vi "Interpolate N Between Two Colors.vi"(0 "Starting Color Value":T1, 2 "# Elements":i32=1 min=1, 3 "Ending Color Value":T1) -> (6 "Color Array":T2(array[cluster]))   [LabVIEW 2021, in "Palette.lvlib"]
uses:
  Palette.lvlib
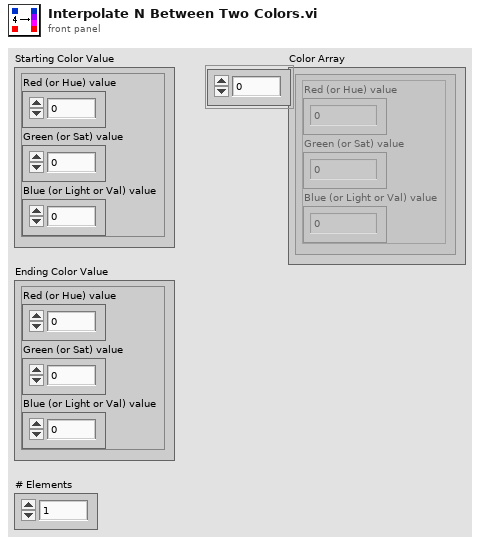
[diagram p1: front panel]
types:
  T1 = cluster{"Red (or Hue) value":u8, "Green (or Sat) value":u8, "Blue (or Light or Val) value":u8}
  T2 = cluster{"Red (or Hue) value":u8, "Green (or Sat) value":u8, "Blue (or Light or Val) value":u8}[]
  T3 = cluster{"Red (or Hue) value":dbl, "Green (or Sat) value":dbl, "Blue (or Light or Val) value":dbl}
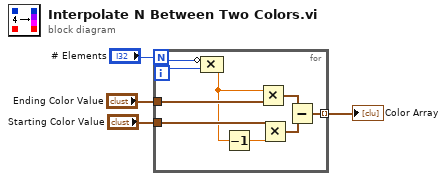
[diagram p0: block diagram]
diagram:
  n1 = for {
    N: "# Elements" -> [w13]
    tunnel: "Ending Color Value" -> [w9]
    tunnel: "Starting Color Value" -> [w10]
    tunnel: [w5] -> w1 mode=indexing
    i -> [w12]
    n2 = Compound Arithmetic op=MULTIPLY(invert w13, w12) -> (w8:dbl)
    n3 = Decrement(x=w8) -> (x-1=w11:dbl)
    n4 = Multiply(x=w8, y=w9) -> (x*y=w7:T3)
    n5 = Multiply(x=w10, y=w11) -> (x*y=w6:T3)
    n6 = Subtract(x=w7, y=w6) -> (x-y=w5:T3)
  }
  "Color Array" <- w1
